vi "LKIF2_SetTiming.vi"(7 "OutNo (OUT1)":T1=1 items=["OUT01"=1, "OUT02"=2, "OUT03"=4, "OUT04"=8, "OUT05"=16, "OUT06"=32, "OUT07"=64, "OUT08"=128, "OUT09"=256, "OUT10"=512, "OUT11"=1024, "OUT12"=2048, "ALL OUT"=4095], 8 "error in (no error)":errorcluster {"code" format="%x"}, 11 "OnOff":bool) -> (0 "error out":errorcluster {"code" format="%x"})   [LabVIEW 2013, in "Keyence LK-G5000.lvlib"]
uses:
  <instrlib>/Keyence LK-G5000/Keyence LK-G5000.lvlib
  <instrlib>/Keyence LK-G5000/Public/enum/LKIF_OUTNO.ctl
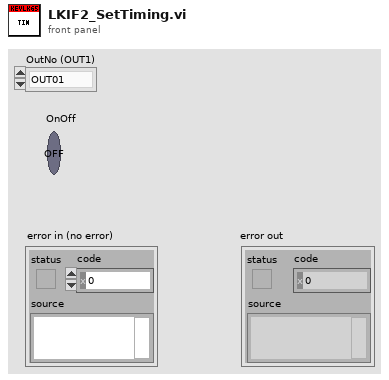
[diagram p1: front panel]
types:
  T1 = typedef "Keyence LK-G5000.lvlib/LKIF_OUTNO.ctl" = i32
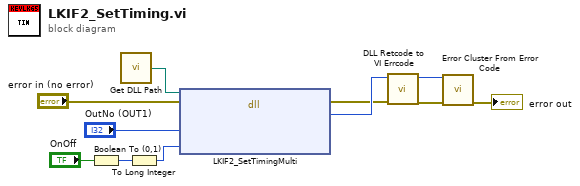
[diagram p0: block diagram]
diagram:
  n1 = Boolean To (0,1)(Boolean="OnOff") -> (0, 1=w6:i16)
  n2 = call <instrlib>:"Get DLL Path.vi"() -> ("DLL Path"=w2:path)  [unwired: 1 in]
  n3 = To Long Integer(number=w6) -> (32bit integer=w5:i32)
  n4 = dll-call lib="C:/Program Files/National Instruments/LabVIEW 2011/instr.lib/Keyence LK-G5000/LKIF2.dll" fn="LKIF2_SetTimingMulti"(path in=w2, error in="error in (no error)", "OutNo"="OutNo (OUT1)", "OnOff"=w5) -> (error out=w3:errorcluster, "RC"=w4:i32)  [unwired: 3 in, 1 out]
  n5 = call <instrlib>:"DLL Retcode to VI Errcode.vi"("error in (no error)"=w3, "DLL Retcode"=w4) -> ("error out"=w11:errorcluster, "VI Errcode"=w10:i32)  [unwired: 8 in]
  n6 = call <vilib>:"Error Cluster From Error Code.vi"("error in (no error)"=w11, "error code (0)"=w10) -> ("error out"=→"error out":errorcluster)  [unwired: 7 in]
